vi "AreArraysIdentical.vi"(5 "ArrayY":i32[](array[numeric]), 6 "ArrayX":i32[](array[numeric])) -> (2 "Equal?":bool)   [LabVIEW 2010]
doc: "This block checks whether or not all of the elements of two I32 arrays are equal, and also checks if the arrays are the same size."
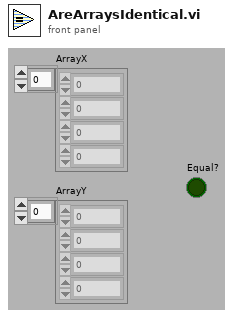
[diagram p1: front panel]
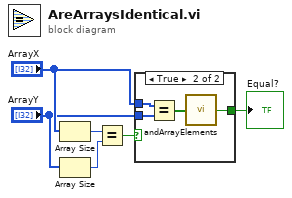
[diagram p0: block diagram]
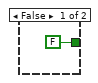
[diagram p2: hidden frame]
diagram:
  n1 = Array Size(array="ArrayX") -> (size(s)=w6:i32)
  n2 = Array Size(array="ArrayY") -> (size(s)=w5:i32)
  n3 = Equal?(x=w6, y=w5) -> (x = y?=w4:bool)
  n4 = case shown="True" w4 {
    tunnel: "ArrayY" -> [_ w11]
    tunnel: "ArrayX" -> [_ w10]
    tunnel: [FALSE w8] -> w1
    frame False {
    }
    frame True {
      n5 = Equal?(x=w10, y=w11) -> (x = y?=w9:bool[])
      n6 = call <vilib>:"andArrayElements.vi"("Boolean Array"=w9) -> ("Logical AND"=w8:bool)
    }
  }
  "Equal?" <- w1
